vi "Main.vi"() -> ()   [LabVIEW 2019]
panel:
  in  "Numeric":i32=100
  out "% Done":dbl
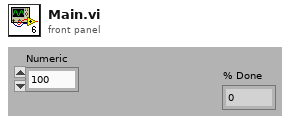
[diagram p1: front panel]
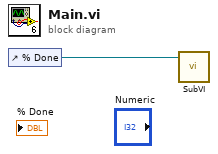
[diagram p0: block diagram]
diagram:
  n1 = control-ref of="% Done"() -> (w1:refnum<vi>)
  n2 = call "SubVI.vi"("% Done Ref"=w1) -> ()  [unwired: 11 in]
